vi "Error.vi"(8 "Error In":errorcluster, 11 "object in":refnum<class "Disconnected.lvclass">) -> (0 "Error Out":errorcluster, 3 "object out":refnum<class "IStates.lvclass">)   [LabVIEW 2023, in "PXI-5441.lvlib" / "Disconnected.lvclass"]
uses:
  Disconnected.lvclass
  IScope_interface/IStates_interface/IStates.lvclass
  Error_class/Error.lvclass
  Disconnected.lvclass/Disconnected.ctl
  D:/git/HAL/PXI-5441_class/states/Error_class/Error.lvclass
  D:/git/HAL/IScope_interface/IStates_interface/IStates.lvclass
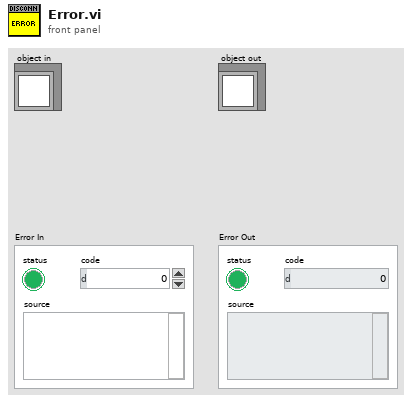
[diagram p1: front panel]
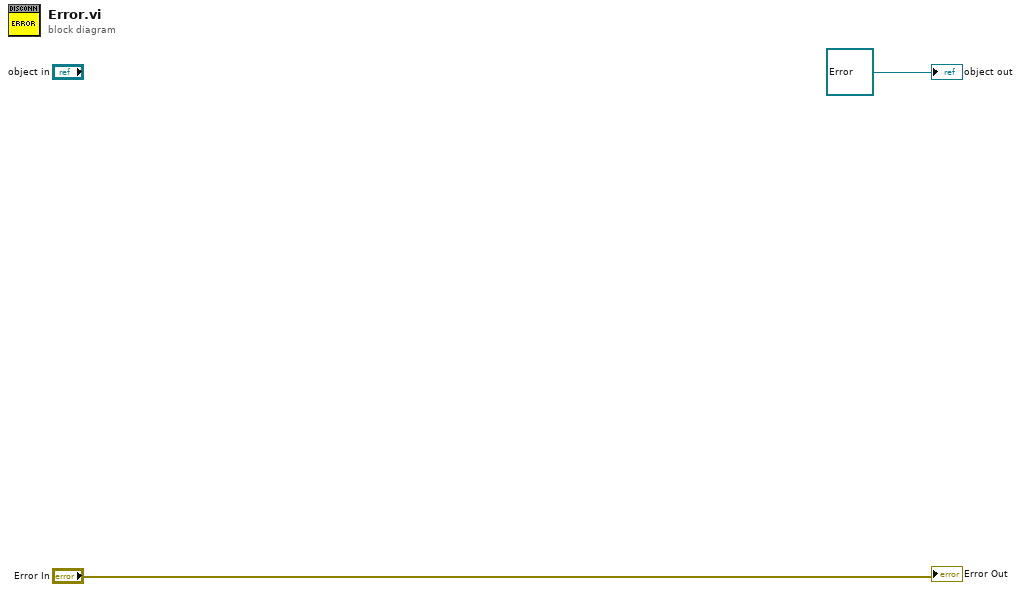
[diagram p0: block diagram]
diagram:
  "Error Out" <- "Error In"
  "object out" <- refnum<class "Error.lvclass"> refnum ("PXI-5441.lvlib:Error")
